vi "Test_image_segmentation.vi"() -> ()   [LabVIEW 2018]
uses:
  <vilib>/Analysis/NI_AAL_Geometry.lvlib
panel:
  in  "Array of points":cluster{"X":dbl, "Y":dbl}[](array[cluster]) {"Y" scale=0.0..640.0; "X" scale=0.0..640.0}
  in  "Stop Button":bool
  out "Image Display":T1(plugin-control)
  out "Error Out":errorcluster
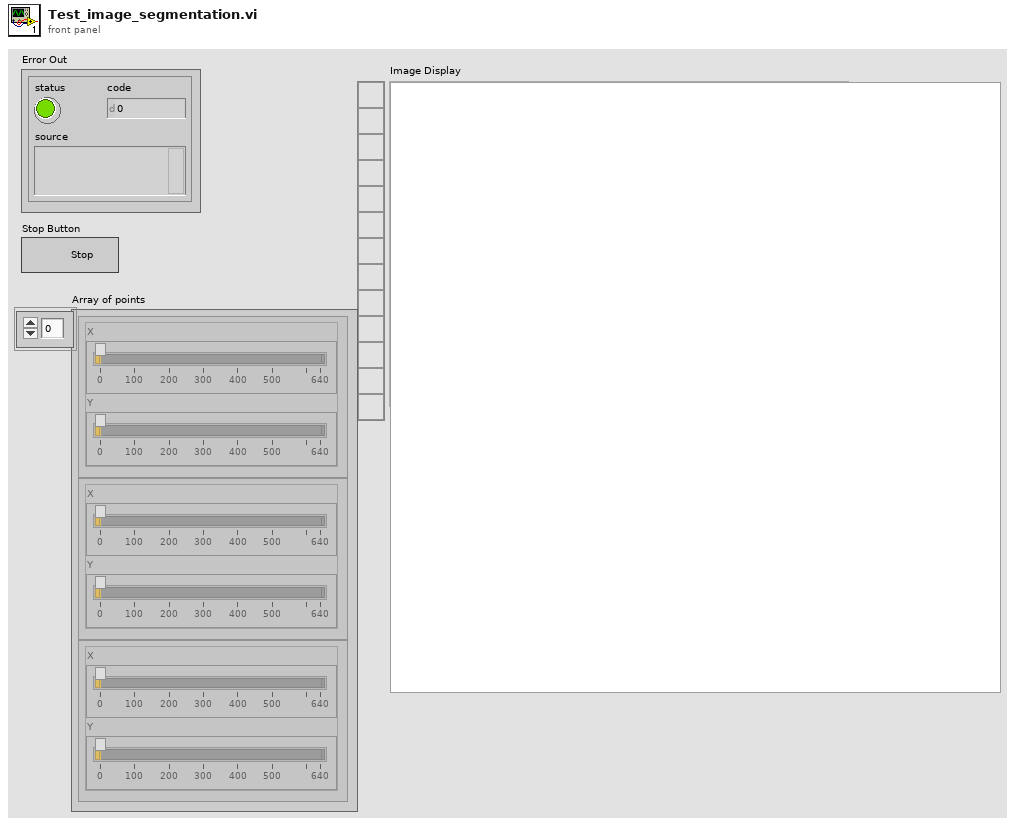
[diagram p1: front panel]
types:
  T1 = typedef "IMAQ Image.ctl" = refnum<image>
  T2 = cluster{"Left":i32, "Top":i32, "Right":i32, "Bottom":i32}
  T3 = typedef "Image Type" = u32
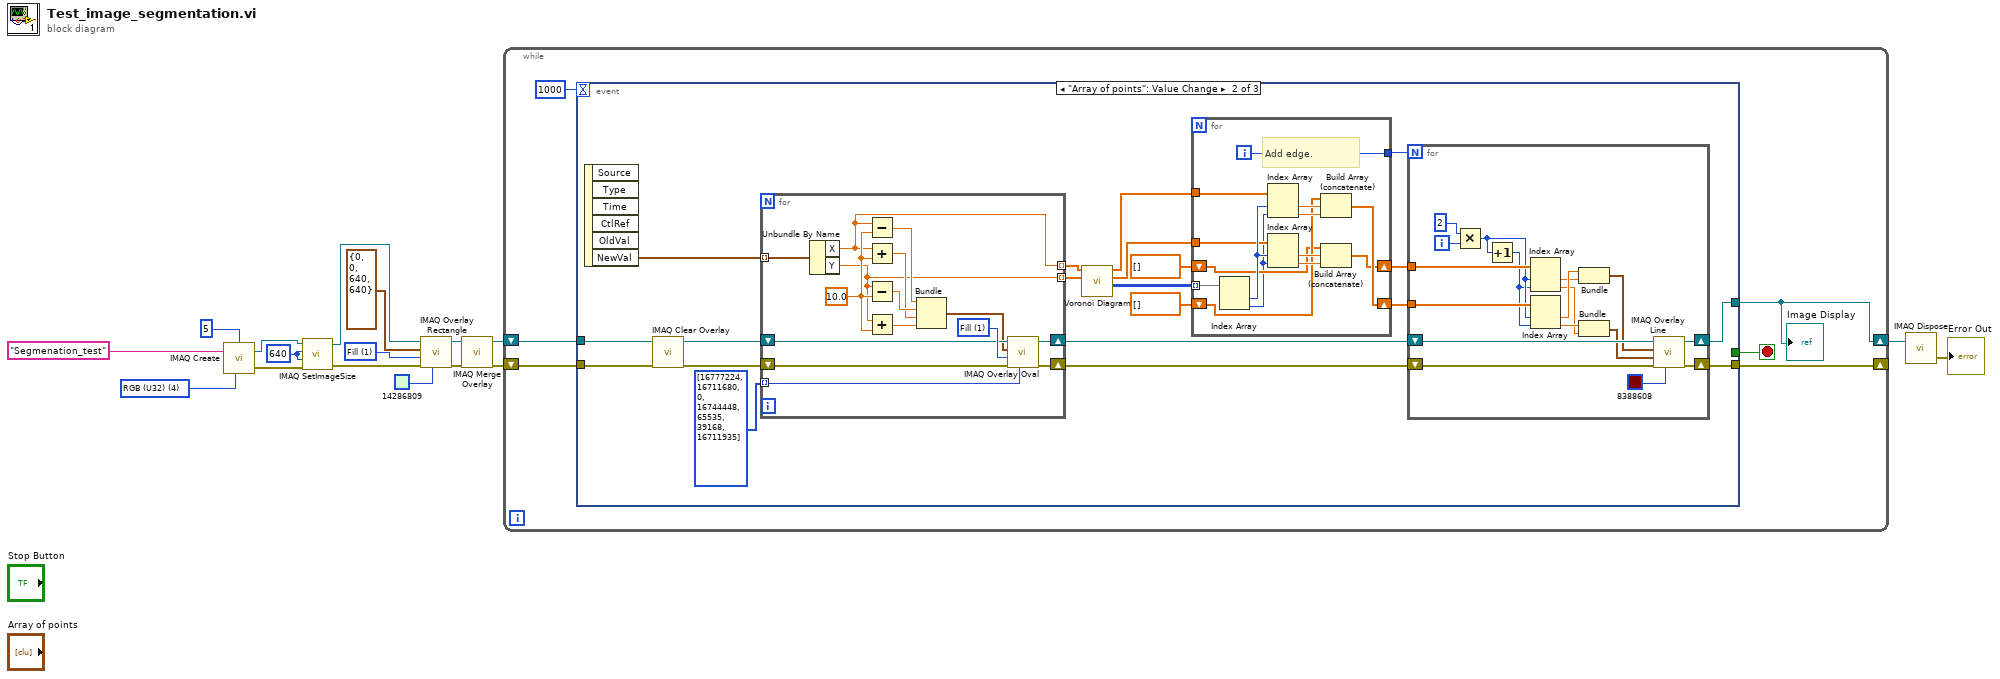
[diagram p0: block diagram]
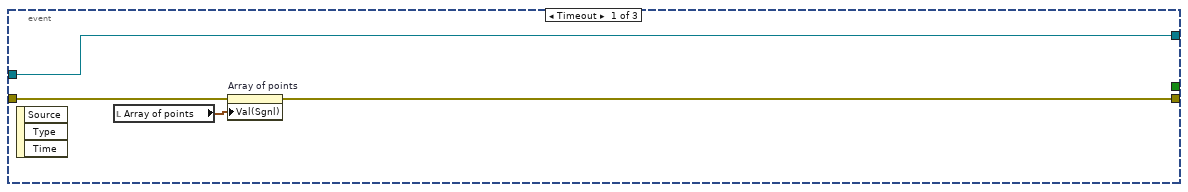
[diagram p2: hidden frame]
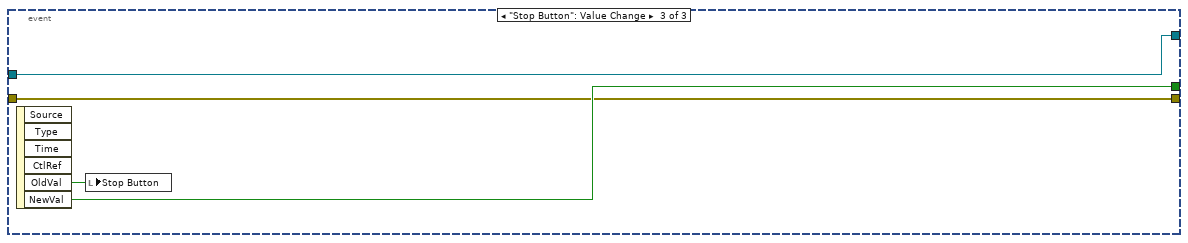
[diagram p3: hidden frame]
diagram:
  w7 = u32 1 items=["Frame", "Fill", "Highlight"] ("Drawing Mode (Frame)")
  w12 = 640 ("X Resolution")
  w16 = T3 4 items=["Grayscale (U8)", "Grayscale (I16)", "Grayscale (SGL)", "Complex (CSG)", "RGB (U32)", "HSL (U32)", "RGB (U64)", "Grayscale (U16)"] ("Image Type")
  n1 = call "IMAQ Create"("Border Size"=5, "Image Name"="Segmenation_test", "Image Type"=w16) -> ("New Image"=w13:T1, "error out"=w14:errorcluster)  [unwired: 2 in]
  n2 = call "IMAQ SetImageSize"("error in (no error)"=w14, "Y Resolution"=w12, "X Resolution"=w12, "Image"=w13) -> ("error out"=w9:errorcluster, "Image Out"=w10:T1)  [unwired: 1 in]
  n3 = call "IMAQ Overlay Rectangle"("Color"=u32 14286809, "error in (no error)"=w9, "Drawing Mode (Frame)"=w7, "Rectangle"=T2 {"Left"=0, "Top"=0, "Right"=640, "Bottom"=640}, "Image"=w10) -> ("error out"=w2:errorcluster, "Image Out"=w4:T1)  [unwired: 5 in]
  n4 = call "IMAQ Merge Overlay"("error in (no error)"=w2, "Image Src"=w4) -> ("error out"=w1:errorcluster, "Image Dst Out"=w3:T1)  [unwired: 8 in]
  n5 = while {
    shift-right: [w21] -> w5
    shift-left: w3 -> [w19]
    shift-right: [w23] -> _
    shift-left: w1 -> [w20]
    stop <- w22 stop-if-true
    n6 = event shown="[1] \"Array of points\": Value Change" {
      selector: _ -> [_ _ _]
      dyn-events: _ -> [_ _ _]
      timeout: 1000 -> [_ _ _]
      tunnel: w19 -> [w27 w46 w95]
      tunnel: [w27 w33 w95] -> w21
      tunnel: [w25 w29 w94] -> w23
      tunnel: [_ _ w96] -> w22
      tunnel: w20 -> [w26 w44 w94]
      event Timeout {
        n7 = event-data() -> ()  [unwired: 1 in, 3 out]
        n8 = local read "Array of points"() -> (w24:cluster{"X":dbl, "Y":dbl}[])
        n9 = property on="Array of points" class="Arr (strict)"(error in=w26, "Val(Sgnl)"=w24) -> (error out=w25:errorcluster)  [unwired: 1 in, 1 out]
      }
      event "Array of points": Value Change {
        n10 = event-data() -> ("NewVal"=w47:cluster{"X":dbl, "Y":dbl}[])  [unwired: 1 in, 5 out]
        n11 = call "IMAQ Clear Overlay"("error in (no error)"=w44, "Image"=w46) -> ("error out"=w43:errorcluster, "Image Out"=w45:T1)  [unwired: 8 in]
        n12 = for {
          tunnel: w47 -> [w93] mode=indexing
          shift-right: [w87] -> w34
          shift-left: w45 -> [w89]
          shift-right: [w88] -> w30
          shift-left: w43 -> [w91]
          tunnel: u32[] [16777224, 16711680, 0, 16744448, 65535, 39168, 16711935] -> [w81] mode=indexing
          tunnel: [w80] -> w36 mode=indexing
          tunnel: [w79] -> w35 mode=indexing
          w90 = u32 1 items=["Frame", "Fill"] ("Drawing Mode (Frame)")
          w86 = 10.0 ("y")
          n13 = Unbundle By Name(w93) -> ("X"=w80:dbl, "Y"=w79:dbl)
          n14 = Subtract(x=w80, y=w86) -> (x-y=w92:dbl)
          n15 = Add(x=w80, y=w86) -> (x+y=w84:dbl)
          n16 = Subtract(x=w79, y=w86) -> (x-y=w85:dbl)
          n17 = Add(x=w79, y=w86) -> (x+y=w83:dbl)
          n18 = Bundle(w92, w85, w84, w83) -> (w82:cluster{dbl, dbl, dbl, dbl})  [unwired: 1 in]
          n19 = call "IMAQ Overlay Oval"("Color"=w81, "error in (no error)"=w91, "Drawing Mode (Frame)"=w90, "Bounding Rectangle"=w82, "Image"=w89) -> ("error out"=w88:errorcluster, "Image Out"=w87:T1)  [unwired: 5 in]
        }
        n20 = call <vilib>:"Voronoi Diagram.vi"("Y"=w35, "X"=w36) -> ("Voronoi Edges"=w41:i32[][], "Voronoi Y"=w37:dbl[], "Voronoi X"=w38:dbl[])  [unwired: 6 in, 1 out]
        n21 = for {
          tunnel: w41 -> [w78] mode=indexing
          shift-right: [w69] -> w32
          shift-left: dbl[] [] -> [w70]
          shift-right: [w67] -> w31
          shift-left: dbl[] [] -> [w68]
          tunnel: w38 -> [w74]
          tunnel: w37 -> [w73]
          tunnel: [w65] -> w28
          i -> [w65]
          # "Add edge."
          n22 = Index Array(array=w78) -> (element #1=w76:i32, element #2=w66:i32)  [unwired: 2 in]
          n23 = Index Array(array=w74, index #1=w76, index #2=w66) -> (element #1=w72:dbl, element #2=w77:dbl)
          n24 = Index Array(array=w73, index #1=w76, index #2=w66) -> (element #1=w71:dbl, element #2=w75:dbl)
          n25 = Build Array (concatenate)(w70, w72, w77) -> (w69:dbl[])
          n26 = Build Array (concatenate)(w68, w71, w75) -> (w67:dbl[])
        }
        n27 = for {
          N: w28 -> [_]
          shift-right: [w61] -> w33
          shift-left: w34 -> [w62]
          tunnel: w32 -> [w64]
          tunnel: w31 -> [w63]
          shift-right: [w59] -> w29
          shift-left: w30 -> [w60]
          i -> [w51]
          n28 = Multiply(x=2, y=w51) -> (x*y=w49:i32)
          n29 = Increment(x=w49) -> (x+1=w48:i32)
          n30 = Index Array(array=w63, index #1=w49, index #2=w48) -> (element #1=w57:dbl, element #2=w54:dbl)
          n31 = Index Array(array=w64, index #1=w49, index #2=w48) -> (element #1=w58:dbl, element #2=w55:dbl)
          n32 = Bundle(w58, "element"=w57) -> (w56:cluster{dbl, "element":dbl})  [unwired: 1 in]
          n33 = Bundle(w55, "element"=w54) -> (w53:cluster{dbl, "element":dbl})  [unwired: 1 in]
          n34 = call "IMAQ Overlay Line"("Color"=u32 8388608, "error in (no error)"=w60, "End Point"=w53, "Start Point"=w56, "Image"=w62) -> ("error out"=w59:errorcluster, "Image Out"=w61:T1)  [unwired: 5 in]
        }
      }
      event "Stop Button": Value Change {
        n35 = event-data() -> ("OldVal"=w97:bool, "NewVal"=w96:bool)  [unwired: 1 in, 4 out]
        n36 = local write "Stop Button"(w97) -> ()
      }
    }
    "Image Display" <- w21
  }
  n37 = call "IMAQ Dispose"("Image"=w5) -> ("error out"=→"Error Out":errorcluster)  [unwired: 5 in]
